vi "ke2002_get_4wR.vi"(8 "error in":errorcluster, 10 "timeout [ms]":i32=5000, 11 "VISA in":refnum<visa-resource-name>) -> (0 "error out":errorcluster, 2 "R value [Ohm]":dbl format="%#_7g", 3 "VISA out":refnum<visa-resource-name>)   [LabVIEW 2020]
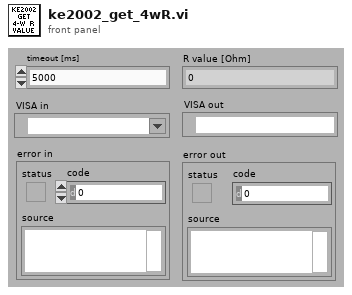
[diagram p1: front panel]
types:
  T1 = cluster{"error":bool, "code":i32, "source":string}
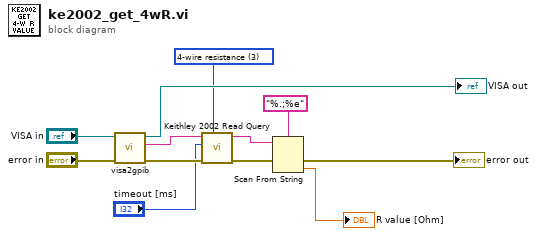
[diagram p0: block diagram]
diagram:
  w8 = u16 3 items=["ac voltage", "dc voltage", "2-wire resistance", "4-wire resistance", "ac current", "dc current", "frequency", "temperature"] ("function (Vdc:1)")
  n1 = call "visa2gpib.vi"("error in"="error in", "VISA in"="VISA in") -> ("error out"=w10:errorcluster, "combined address"=w3:string, "VISA out"=→"VISA out":refnum<visa-resource-name>)  [unwired: 7 in]
  n2 = call "Keithley 2002 Read Query.vi"("function (Vdc:1)"=w8, "error in"=w10, "timeout ms"="timeout [ms]", "GPIB Address"=w3) -> ("error out"=w7:T1, "Reading Result"=w5:string)  [unwired: 6 in]
  n3 = Scan From String(format string="%.;%e", input string=w5, error in=w7) -> (error out=→"error out":errorcluster, output 1=→"R value [Ohm]":dbl)  [unwired: 2 in, 2 out]
